vi "Write DMA adresses.vi"(8 "error in (no error)":errorcluster, 10 "DMA adresses":i64[](array[numeric]), 11 "Config params in":refnum<class "CV-Configuration.lvclass">) -> (0 "error out":errorcluster, 3 "Config params out":refnum<class "CV-Configuration.lvclass">)   [LabVIEW 2013, in "CameraVision.lvlib" / "CV-Configuration.lvclass"]
uses:
  CV-Configuration.lvclass
  CV-Configuration.lvclass/CV-Configuration.ctl
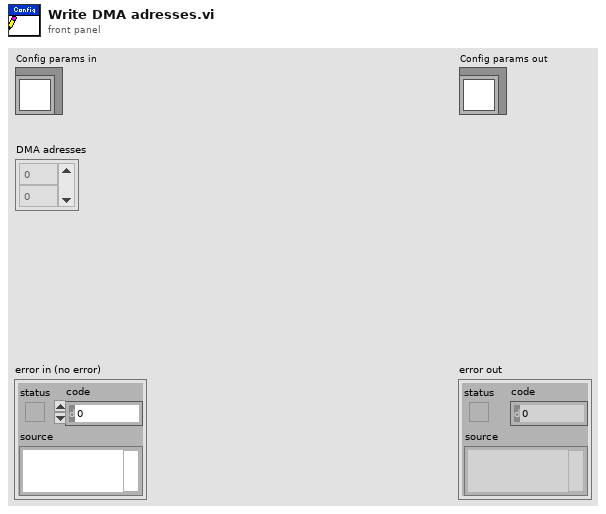
[diagram p1: front panel]
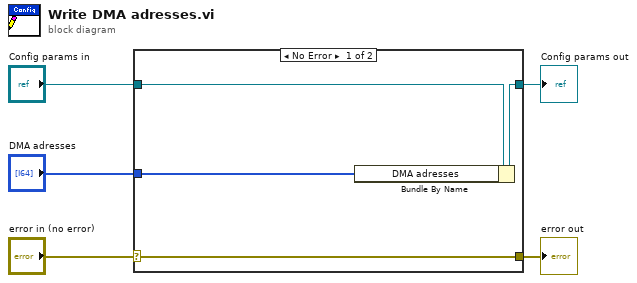
[diagram p0: block diagram]
diagram:
  n1 = case shown="No Error" "error in (no error)" {
    selector: "error in (no error)" -> [w9 w10]
    tunnel: [w9 w10] -> w4
    tunnel: [w7 w11] -> w2
    tunnel: "Config params in" -> [w8 w11]
    tunnel: "DMA adresses" -> [w6 _]
    frame No Error {
      n2 = Bundle By Name(cluster=w8, "DMA adresses"=w6) -> (w7:refnum<class "CV-Configuration.lvclass">)
    }
    frame Error {
    }
  }
  "error out" <- w4
  "Config params out" <- w2
